vi "Close FPGA Reference.vi"(8 "error in (no error)":errorcluster, 11 "Data in":T1) -> (0 "error out":errorcluster)   [LabVIEW 2017, in "Test Bench.lvlib"]
uses:
  Test Bench.lvlib
  Scan Engine Variables.ctl
  <instrlib>/_niInstr/FIFO Register Bus/v1/Host/niInstr FIFO Register Bus v1 Host.lvclass
  <instrlib>/_niInstr/Instruction Framework/v1/Host/Instruction Framework Context/niInstr Instruction Framework Context v1 Host.lvclass
  <vilib>/FPGAPlugInAG/Dynamic/niLvFpga_Close_Dynamic.vi
  <vilib>/rvi/interface/nirviCloseFPGA/nirviCloseFPGA.xnode
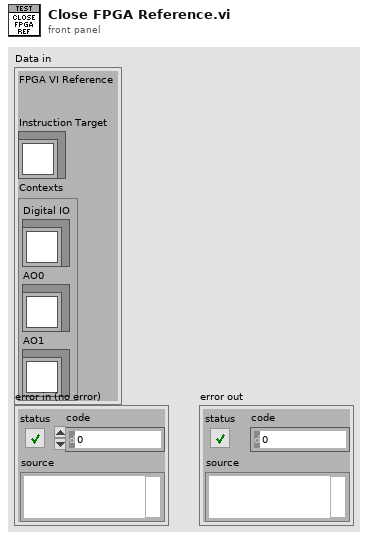
[diagram p1: front panel]
types:
  T1 = typedef "Test Bench.lvlib/Scan Engine Variables.ctl" = cluster{"FPGA VI Reference":refnum<k20>, "Instruction Target":refnum<class "niInstr FIFO Register Bus v1 Host.lvclass">, "Contexts":cluster{"Digital IO":refnum<class "niInstr Instruction Framework Context v1 Host.lvclass">, "AO0":refnum<class "niInstr Instruction Framework Context v1 Host.lvclass">, "AO1":refnum<class "niInstr Instruction Framework Context v1 Host.lvclass">}}
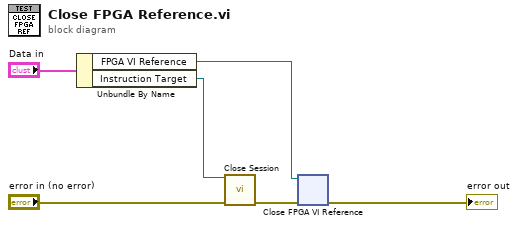
[diagram p0: block diagram]
diagram:
  n1 = Unbundle By Name("Data in") -> ("FPGA VI Reference"=w4:refnum<k20>, "Instruction Target"=w3:refnum<class "niInstr FIFO Register Bus v1 Host.lvclass">)
  n2 = call-dynamic "Close Session.vi"("session in"=w3, "error in"="error in (no error)") -> ("error out"=w6:errorcluster)  [unwired: 13 in]
  n3 = xnode "Close FPGA VI Reference"("FPGA VI Reference In"=w4, "error in"=w6) -> ("error out"=→"error out":errorcluster)
